vi "SaveFile.vi"(6 "Header":string, 7 "Average FRF in":cluster{"x0":dbl, "df":dbl, dbl[]}, 9 "i":i32, 10 "filename":string, 11 "Folder":path) -> (2 "Y":cdb[](array[numeric]), 3 "Header Info":T1)   [LabVIEW 2024]
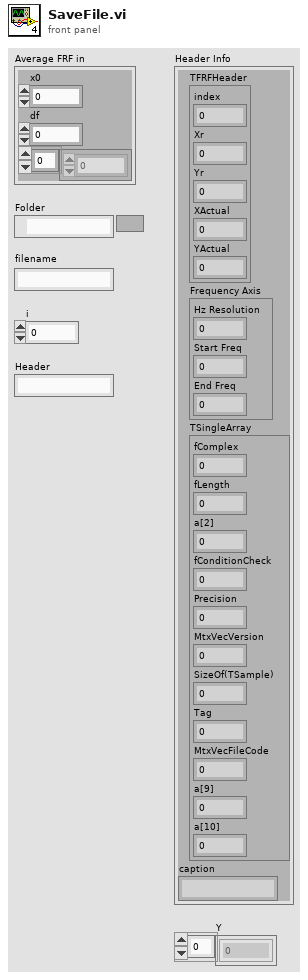
[diagram p1: front panel]
types:
  T1 = cluster{"TFRFHeader":cluster{"index":u32, "Xr":dbl, "Yr":dbl, "XActual":dbl, "YActual":dbl}, "Frequency Axis":cluster{"Hz Resolution":dbl, "Start Freq":dbl, "End Freq":dbl}, "TSingleArray":cluster{"fComplex":u32, "fLength":dbl, "a[2]":dbl, "fConditionCheck":dbl, "Precision":dbl, "MtxVecVersion":dbl, "SizeOf(TSample)":dbl, "Tag":dbl, "MtxVecFileCode":dbl, "a[9]":dbl, "a[10]":dbl}, "caption":string}
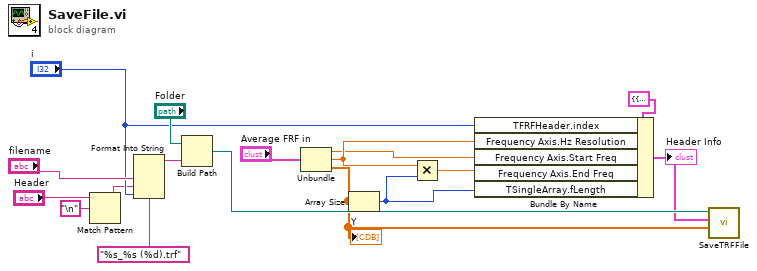
[diagram p0: block diagram]
diagram:
  n1 = Match Pattern(string="Header", regular expression="\n") -> (before substring=w1:string)  [unwired: 1 in, 3 out]
  n2 = Format Into String(format string="%s_%s (%d).trf", "filename", w1, "i") -> (resulting string=w2:string)  [unwired: 2 in, 1 out]
  n3 = Build Path(base path="Folder", name or relative path=w2) -> (appended path=w17:path)
  n4 = Unbundle("Average FRF in") -> ("x0"=w9:dbl, "df"=w11:dbl, w16:dbl[])
  "Y" <- w16
  n5 = Array Size(array=w16) -> (size(s)=w10:i32)
  n6 = Multiply(x=w11, y=w10) -> (x*y=w12:dbl)
  n7 = Bundle By Name(cluster=T1 {"TFRFHeader"={"index"=11, "Xr"=0.0, "Yr"=0.0, "XActual"=0.0, "YActual"=0.0}, "Frequency Axis"={"Hz Resolution"=0.732421875, "Start Freq"=199.951171875, "End Freq"=9999.755859375}, "TSingleArray"={"fComplex"=1, "fLength"=13381.0, "a[2]"=0.0, "fConditionCheck"=1.0, "Precision"=0.0, "MtxVecVersion"=420.0, "SizeOf(TSample)"=8.0, "Tag"=0.0, "MtxVecFileCode"=64019.0, "a[9]"=0.0, "a[10]"=0.0}, "caption"="\u0000\u0000\u0000\u0000"} ("Header Info"), "TFRFHeader.index"="i", "Frequency Axis.Hz Resolution"=w11, "Frequency Axis.Start Freq"=w9, "Frequency Axis.End Freq"=w12, "TSingleArray.fLength"=w10) -> (w15:T1)
  "Header Info" <- w15
  n8 = call "SaveTRFFile.vi"("Y"=w16, "Header Info"=w15, "trf file in"=w17) -> ()  [unwired: 7 in, 2 out]
